vi "Wago PLC.vi"(8 "error in (no error)":errorcluster) -> (0 "error out":errorcluster)   [LabVIEW 2021]
uses:
  <vilib>/Modbus/slave/Create Slave Instance (TCP).vi
  <vilib>/Modbus/slave/Modbus Slave.lvclass
panel:
  in  "error in (no error) 2":errorcluster
  in  "Array":dbl[](array[numeric])
  out "output array":sgl[](array[numeric])
  in  "Array 3":sgl[](array[numeric]) format="%#_7g"
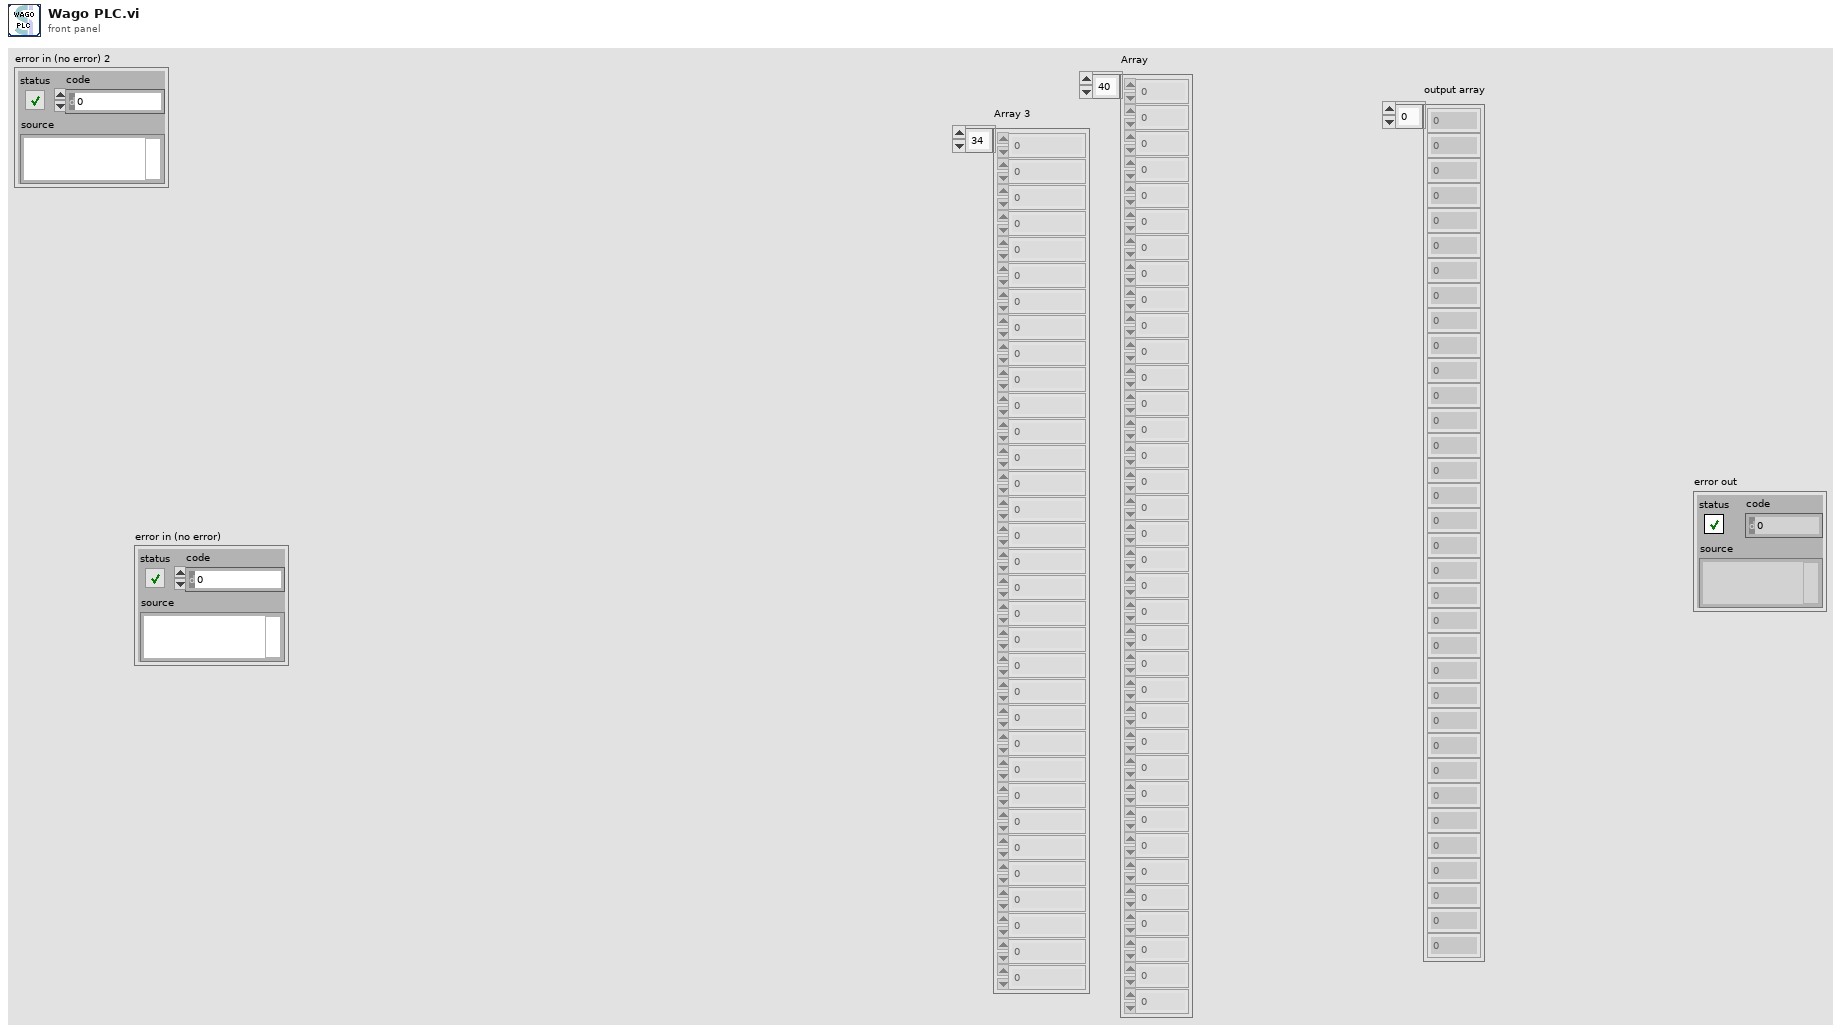
[diagram p1: front panel]
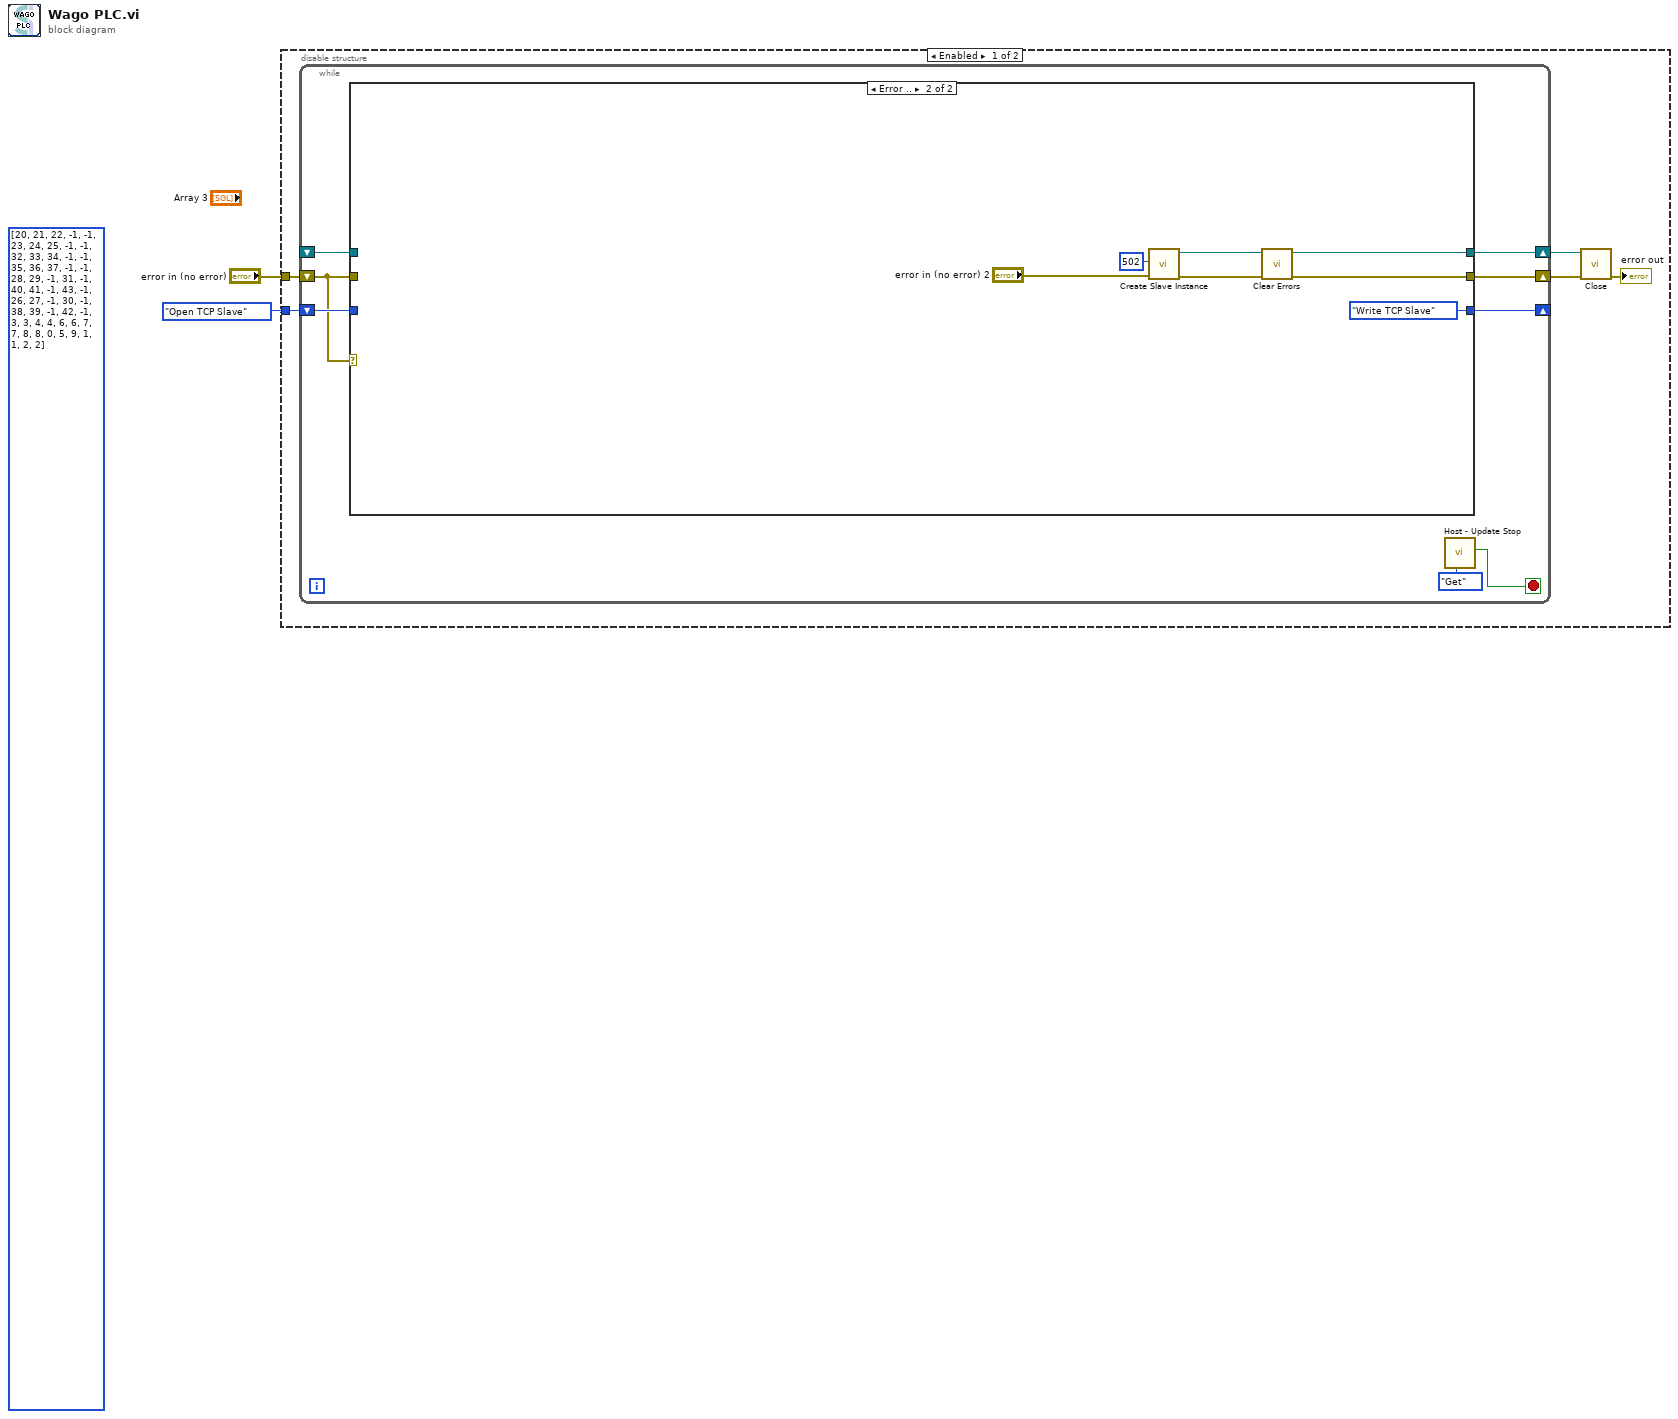
[diagram p0: block diagram]
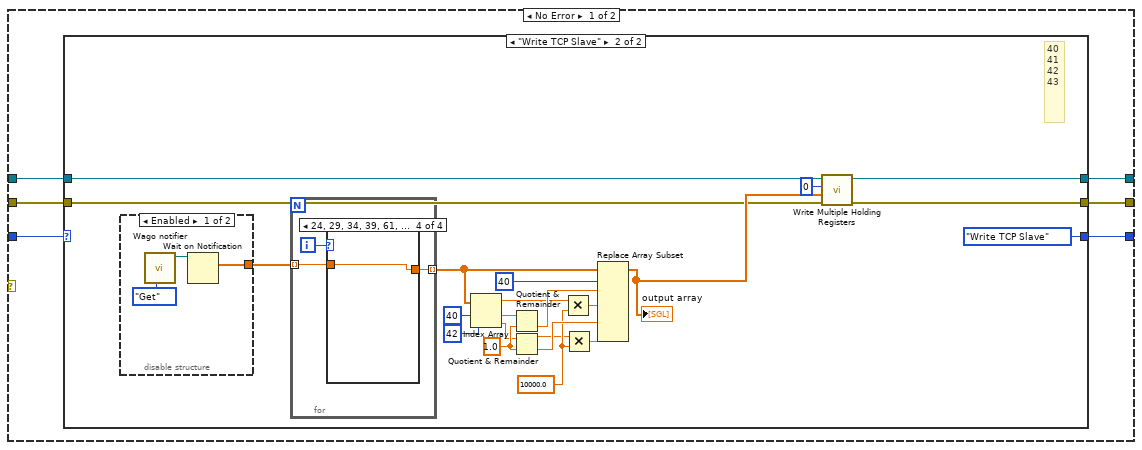
[diagram p2: hidden frame]
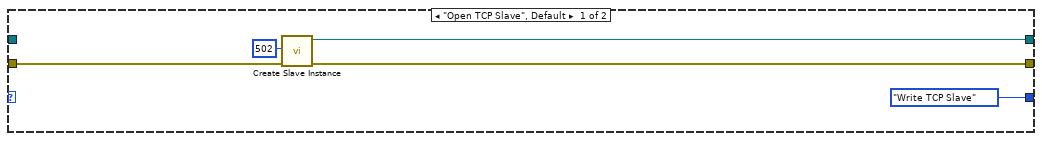
[diagram p3: hidden frame]
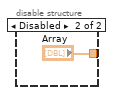
[diagram p4: hidden frame]
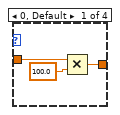
[diagram p5: hidden frame]
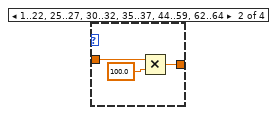
[diagram p6: hidden frame]
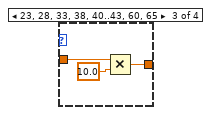
[diagram p7: hidden frame]
diagram:
  (unwired) i32[] [20, 21, 22, -1, -1, 23, 24, 25, -1, -1, 32, 33, 34, -1, -1, 35, 36, 37, -1, -1, 28, 29, -1, 31, -1, 40, 41, -1, 43, -1, 26, 27, -1, 30, -1, 38, 39, -1, 42, -1, 3, 3, 4, 4, 6, 6, 7, 7, 8, 8, 0, 5, 9, 1, 1, 2, 2]
  n1 = disable-structure shown="Enabled" {
    disable-tunnel: "error in (no error)" -> [w3 _]
    disable-tunnel: enum16{"Open TCP Slave", "Write TCP Slave"}."Open TCP Slave" ("Enum") -> [w4 _]
    frame Enabled {
      n2 = while {
        shift-right: [w14] -> w5
        shift-left: _ -> [w12]
        shift-right: [w11] -> _
        shift-left: w4 -> [w13]
        shift-right: [w15] -> w6
        shift-left: w3 -> [w8]
        stop <- w9 stop-if-true
        n3 = case shown="Error .." w8 {
          tunnel: w8 -> [w21 _]
          tunnel: [w20 w67] -> w15
          tunnel: [w19 w69] -> w14
          tunnel: w13 -> [w18 _]
          tunnel: w12 -> [w17 _]
          tunnel: [w16 enum16{"Open TCP Slave", "Write TCP Slave"}."Write TCP Slave" ("Enum")] -> w11
          frame No Error {
            n4 = case shown="\"Write TCP Slave\"" w18 {
              tunnel: w21 -> [w25 w32]
              tunnel: [w23 w30] -> w20
              tunnel: [w24 w29] -> w19
              tunnel: w17 -> [_ w28]
              tunnel: [enum16{"Open TCP Slave", "Write TCP Slave"}."Write TCP Slave" ("Enum") enum16{"Open TCP Slave", "Write TCP Slave"}."Write TCP Slave" ("Enum")] -> w16
              frame "Open TCP Slave", Default {
                n5 = call-poly <vilib>:"Create Slave Instance.vi"("error in (no error)"=w25, "port (502)"=u16 502) -> ("error out"=w23:errorcluster, "TCP slave instance"=w24:refnum<class "Modbus Slave.lvclass">)  [unwired: 8 in]
              }
              frame "Write TCP Slave" {
                w37 = 10000.0 ("y")
                w44 = sgl 1.0 ("y")
                # "40\n41\n42\n43"
                n6 = disable-structure shown="Enabled" {
                  disable-tunnel: [w49 "Array"] -> w33
                  frame Enabled {
                    n7 = call "Wago notifier.vi"("Operation"=enum16{"Init", "Get", "Set"}."Get") -> ("notifier out"=w50:refnum<notifier>)  [unwired: 9 in, 1 out]
                    n8 = Wait on Notification(notifier=w50) -> (notification=w49:sgl[])  [unwired: 3 in, 3 out]
                  }
                  frame Disabled {
                  }
                }
                n9 = for {
                  tunnel: w33 -> [w53] mode=indexing
                  tunnel: [w55] -> w46 mode=indexing
                  i -> [w54]
                  n10 = case shown="24, 29, 34, 39, 61, 66" w54 {
                    tunnel: w53 -> [w58 w60 w64 w65]
                    tunnel: [w56 w59 w62 w65] -> w55
                    frame 0, Default {
                      n11 = Multiply(x=w58, y=sgl 100.0) -> (x*y=w56:sgl)
                    }
                    frame 1..22, 25..27, 30..32, 35..37, 44..59, 62..64 {
                      n12 = Multiply(x=w60, y=sgl 100.0) -> (x*y=w59:sgl)
                    }
                    frame 23, 28, 33, 38, 40..43, 60, 65 {
                      n13 = Multiply(x=w64, y=sgl 10.0) -> (x*y=w62:sgl)
                    }
                    frame 24, 29, 34, 39, 61, 66 {
                    }
                  }
                }
                n14 = Index Array(array=w46, index #1=40 ("index"), index #2=42 ("index")) -> (element #1=w45:sgl, element #2=w43:sgl)
                n15 = Quotient & Remainder(x=w45, y=w44) -> (x-y*floor(x/y)=w40:sgl, floor(x/y)=w41:sgl)
                n16 = Quotient & Remainder(x=w43, y=w44) -> (x-y*floor(x/y)=w36:sgl, floor(x/y)=w38:sgl)
                n17 = Multiply(x=w40, y=w37) -> (x*y=w39:dbl)
                n18 = Multiply(x=w36, y=w37) -> (x*y=w35:dbl)
                n19 = Replace Array Subset "Replace Array Subset"(array=w46, new element #1=w41, index #1=40 ("index"), new element #2=w39, new element #3=w38, new element #4=w35) -> (w34:sgl[])  [unwired: 3 in]
                "output array" <- w34
                n20 = call-dynamic "Write Multiple Holding Registers.vi"("error in (no error)"=w32, "holding register values"=w34, "starting address"=u16 0, "Modbus slave in"=w28) -> ("error out"=w30:errorcluster, "Modbus slave out"=w29:refnum<class "Modbus Slave.lvclass">)  [unwired: 6 in]
              }
            }
          }
          frame Error {
            n21 = call-poly <vilib>:"Create Slave Instance.vi"("error in (no error)"="error in (no error) 2", "port (502)"=u16 502) -> ("error out"=w68:errorcluster, "TCP slave instance"=w69:refnum<class "Modbus Slave.lvclass">)  [unwired: 8 in]
            n22 = call <vilib>:"Clear Errors.vi"("error in (no error)"=w68) -> ("error out"=w67:errorcluster)  [unwired: 5 in, 1 out]
          }
        }
        n23 = call "Host - Update Stop.vi"("Operation"=enum16{"Init", "Get", "Set"}."Get") -> ("Stop?"=w9:bool)  [unwired: 9 in, 1 out]
      }
      n24 = call-dynamic "Close.vi"("error in (no error)"=w6, "Modbus slave in"=w5) -> ("error out"=→"error out":errorcluster)  [unwired: 9 in]
    }
    frame Disabled {
    }
  }
